vi "PH_AWG-510.constructor.vi"(0 "name":string, 2 "data in":string, 5 "error in":errorcluster) -> (14 "i ref out":refnum<vi>, 16 "data out":string, 19 "error out":errorcluster)   [LabVIEW 2014, in "PH_AWG-510.lvlib"]
doc: "AWG 510\n\nauthor: Stefan Götte, PHELIX\n\nLicense Agreement for this software:\n\nCopyright (C)\nGesellschaft für Schwerionenforschung, GSI\nPlanckstr. 1\n64291 Darmstadt\nGermany\n\nContact: D.Beck@gsi.de \n\nThis program is free software; you can redistribute it and/or modify it under the terms of the \nGNU General Public License as published by the Free Software Foundation; either version 2 of \nthe license, or (at your option) any later version.\n\nThis program is distributed in the hope that it will be useful, but WITHOUT ANY WARRANTY; \nwithout even the implied warranty of MERCHANTABILITY or FITNESS FOR A PARTICULAR PURPOSE. See the GNU General License for more details (http://www.gnu.org).\n\nGesellschaft für Schwerionenforschung, GSI\nPlanckstr. 1, 64291 Darmstadt, Germany\nFor all questions and ideas contact: M.Richter@gsi.de, H.Brand@gsi.de or D.Beck@gsi.de.\nLast update: 16-JUN-2004"
uses:
  PH_AWG-510.lvlib
  PH_PSDBWriter/PH_PSDBWriter.lvlib
  PH_Class/PH_Class.lvlib
  PH_StatusHandler/PH_StatusHandler.lvlib
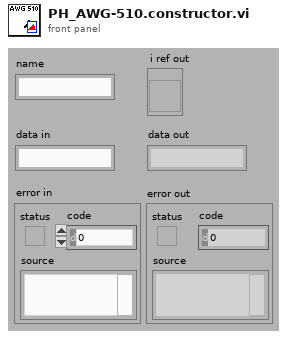
[diagram p1: front panel]
types:
  T1 = enum16{"SetAttribute", "GetAttribute", "CreateAttribute", "DestroyAttribute", "DestroyAllAtributes"}
  T2 = typedef "PH_AWG-510.lvlib/PH_AWG-510.i attribute.ctl" = cluster{"GUI Refs":cluster{"Delete":refnum<vi>, "Trigger Settings":refnum<vi>, "Start Device":refnum<vi>, "Instrument Information":refnum<vi>, "Lock Frontpanel":refnum<vi>, "Waveform Pattern File":refnum<vi>, "Initialize":refnum<vi>, "Output Settings":refnum<vi>}, "Instrument Information":T3, "Initialized?":bool, "Current Settings":cluster{"Trigger":T4, "Output Settings":T5}, "Wanted Settings":cluster{"Trigger":T4, "Output Settings":T5}, "Device frontpanel locked?":bool, "Default File Path":path}
  T3 = typedef "PH_AWG-510.lvlib/PH_AWG-510.Instrument Information Dataset.ctl" = cluster{"VISA resource name":refnum<visa-resource-name>, "Instrument Firmware Revision":string, "Manufacturer":string, "Model":string, "Serial Number":string, "Error Message":string, "Device Status":enum16{"stopped", "wating for trigger", "running", "Failure"}}
  T4 = typedef "PH_AWG-510.lvlib/PH_AWG-510.Trigger Settings.ctl" = cluster{"Mode":enum16{"Continuous", "Triggered", "Gated", "Enhanced"}, "Level (V)":dbl, "External Source":bool}
  T5 = typedef "PH_AWG-510.lvlib/PH_AWG-510.Output Settings.ctl" = cluster{"Activate Channel":bool, "VPP (V)":dbl, "Clock (Hz)":dbl, "File Name (Device)":string, "#1":u16, "#2":u16, "#3":u16, "#4":u16, "#5":u16, "#6":u16, "#7":u16, "#8":u16, "#9":u16, "#10":u16, "#11":u16, "#12":u16, "#13":u16, "#14":u16, "#15":u16, "#16":u16, "#17":u16, "#18":u16, "#19":u16, "#20":u16, "Offset (V)":dbl}
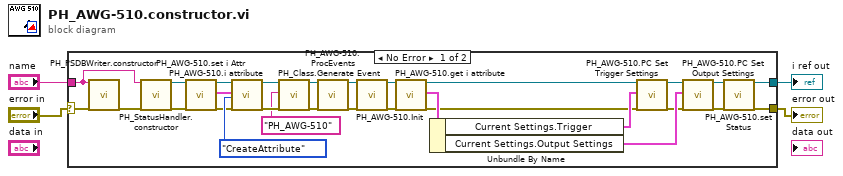
[diagram p0: block diagram]
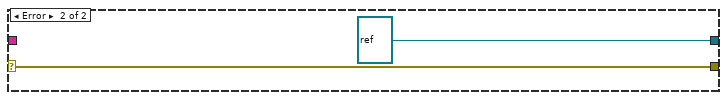
[diagram p2: hidden frame]
diagram:
  n1 = case shown="No Error" "error in" {
    selector: "error in" -> [w12 w34]
    tunnel: "name" -> [w5 _]
    tunnel: [w19 w34] -> w3
    tunnel: [w20 refnum<vi> refnum ("i ref out")] -> w2
    frame No Error {
      n2 = call "PH_PSDBWriter.constructor.vi"("name"=w5, "error in"=w12) -> ("error out"=w11:errorcluster)  [unwired: 15 in, 2 out]
      n3 = call "PH_StatusHandler.constructor.vi"("name"=w5, "error in(no error)"=w11) -> ("i ref out"=w6:refnum<vi>, "error out"=w7:errorcluster)  [unwired: 15 in, 1 out]
      n4 = call "PH_AWG-510.set i Attr.vi"("i ref in"=w6, "error in"=w7) -> ("i ref out"=w9:refnum<vi>, "i Attributes"=w10:T2, "error out"=w8:errorcluster)  [unwired: 15 in]
      n5 = call "PH_AWG-510.i attribute.vi"("VI Refnum"=w9, "CLASS.i attribute"=w10, "Action"=T1."CreateAttribute", "error in (no error)"=w8) -> ("VI Refnum out"=w15:refnum<vi>, "error out"=w14:errorcluster)  [unwired: 13 in, 1 out]
      n6 = call "PH_Class.Generate Event.vi"("i ref in"=w15, "Class"="PH_AWG-510", "error in (no error)"=w14) -> ("i ref out"=w17:refnum<vi>, "error out"=w16:errorcluster)  [unwired: 15 in]
      n7 = call "PH_AWG-510.ProcEvents.vi"("i ref in"=w17, "error in"=w16) -> ("i ref out"=w22:refnum<vi>, "error out"=w21:errorcluster)  [unwired: 16 in]
      n8 = call "PH_AWG-510.Init.vi"("VI in"=w22, "error in (no error)"=w21) -> ("VI out"=w23:refnum<vi>, "error out"=w24:errorcluster)  [unwired: 16 in]
      n9 = call "PH_AWG-510.get i attribute.vi"("i ref in"=w23, "error in (no error)"=w24) -> ("i ref out"=w27:refnum<vi>, "i attribute"=w28:T2, "error out"=w25:errorcluster)  [unwired: 15 in]
      n10 = Unbundle By Name(w28) -> ("Current Settings.Trigger"=w29:T4, "Current Settings.Output Settings"=w33:T5)
      n11 = call "PH_AWG-510.PC Set Trigger Settings.vi"("VI in"=w27, "Wanted Trigger Settings"=w29, "error in (no error)"=w25) -> ("VI out"=w31:refnum<vi>, "error out"=w26:errorcluster)  [unwired: 15 in]
      n12 = call "PH_AWG-510.PC Set Output Settings.vi"("VI in"=w31, "Wanted Output Settings"=w33, "error in (no error)"=w26) -> ("VI out"=w32:refnum<vi>, "error out"=w30:errorcluster)  [unwired: 15 in]
      n13 = call "PH_AWG-510.set Status.vi"("i ref in"=w32, "error in"=w30) -> ("i ref out"=w20:refnum<vi>, "error out"=w19:errorcluster)  [unwired: 16 in]
    }
    frame Error {
    }
  }
  "i ref out" <- w2
  "error out" <- w3
